vi "MGCC_StaEst_initial_input_RTDS.vi"() -> ()   [LabVIEW 2016]
doc: "-----------------------------------------------------------------------------------------------------------------------\nCopyright <2019> <The University of Tennessee at Knoxville and the University of Tennessee Research Foundation>\nThis software is released under BSD-3 \nhttps://opensource.org/licenses/BSD-3-Clause \nAdditional license options available at https://utrf.tennessee.edu/industry/sample-agreements/\n-----------------------------------------------------------------------------------------------------------------------"
uses:
  <vilib>/Utility/error.llb/Error Cluster From Error Code.vi
  <vilib>/ErrorRing/Error Ring.xnode
panel:
  out "element":i32
  out "size(s)":i32[](array[numeric])
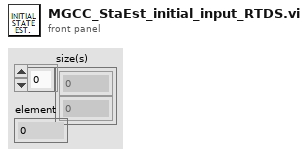
[diagram p1: front panel]
types:
  T1 = cluster{"V_node":cdb[][], "P_node":cdb[][], "I_node":cdb[][], "NumN":dbl, "NumL":dbl, "Ybus":cdb[][], "sspn":dbl[][], "ssqn":dbl[][], "ssvn":dbl[][], "SlackBus":dbl, "Topology":dbl[][]}
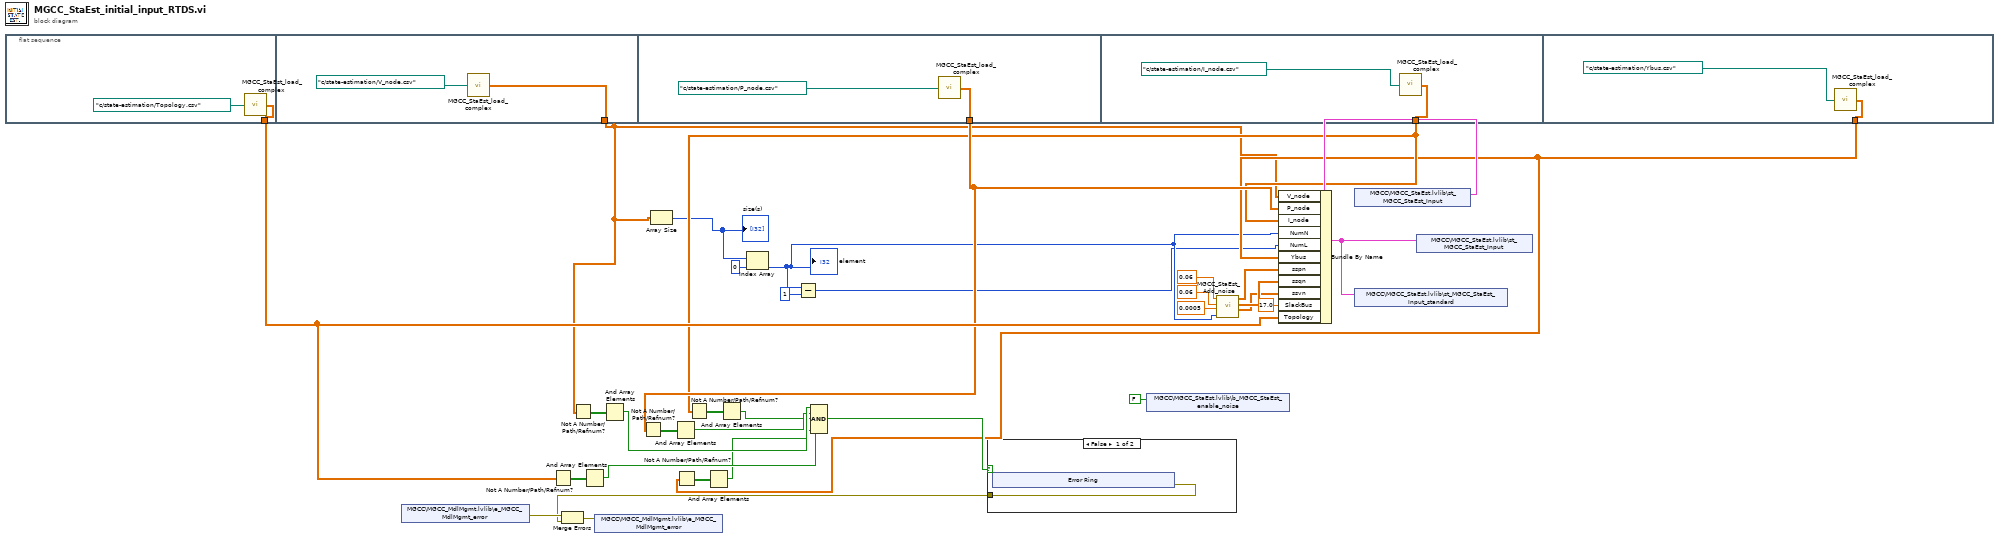
[diagram p0: block diagram]
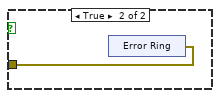
[diagram p2: hidden frame]
diagram:
  n1 = flat-sequence {
    tunnel: [w35] -> w12
    tunnel: [w37] -> w6
    tunnel: [w39] -> w11
    tunnel: [w41] -> w10
    tunnel: [w43] -> w8
    frame #0 {
      n2 = call "MGCC_StaEst_load_complex.vi"("file path (dialog if empty)"=path "c:/state-estimation/Topology.csv" ("file path (use dialog)")) -> ("Array 13"=w35:cdb[][])
    }
    frame #1 {
      n3 = call "MGCC_StaEst_load_complex.vi"("file path (dialog if empty)"=path "c:/state-estimation/V_node.csv" ("file path (use dialog)")) -> ("Array 13"=w37:cdb[][])
    }
    frame #2 {
      n4 = call "MGCC_StaEst_load_complex.vi"("file path (dialog if empty)"=path "c:/state-estimation/P_node.csv" ("file path (use dialog)")) -> ("Array 13"=w39:cdb[][])
    }
    frame #3 {
      n5 = call "MGCC_StaEst_load_complex.vi"("file path (dialog if empty)"=path "c:/state-estimation/I_node.csv" ("file path (use dialog)")) -> ("Array 13"=w41:cdb[][])
    }
    frame #4 {
      n6 = call "MGCC_StaEst_load_complex.vi"("file path (dialog if empty)"=path "c:/state-estimation/Ybus.csv" ("file path (use dialog)")) -> ("Array 13"=w43:cdb[][])
    }
  }
  n7 = shared-variable "MGCC\\MGCC_MdlMgmt.lvlib\\e_MGCC_MdlMgmt_error"() -> (w24:errorcluster)  [unwired: 1 in, 1 out]
  n8 = Not A Number/Path/Refnum?(number/path/refnum=w12) -> (NaN/Path/Refnum?=w21:bool[][])
  n9 = Not A Number/Path/Refnum?(number/path/refnum=w6) -> (NaN/Path/Refnum?=w20:bool[][])
  n10 = And Array Elements(Boolean array=w21) -> (logical AND=w14:bool)
  n11 = And Array Elements(Boolean array=w20) -> (logical AND=w17:bool)
  n12 = Not A Number/Path/Refnum?(number/path/refnum=w11) -> (NaN/Path/Refnum?=w18:bool[][])
  n13 = Array Size(array=w6) -> (size(s)=w5:i32[])
  "size(s)" <- w5
  n14 = And Array Elements(Boolean array=w18) -> (logical AND=w16:bool)
  n15 = Not A Number/Path/Refnum?(number/path/refnum=w8) -> (NaN/Path/Refnum?=w9:bool[][])
  n16 = Not A Number/Path/Refnum?(number/path/refnum=w10) -> (NaN/Path/Refnum?=w19:bool[][])
  n17 = And Array Elements(Boolean array=w9) -> (logical AND=w7:bool)
  n18 = And Array Elements(Boolean array=w19) -> (logical AND=w15:bool)
  n19 = Index Array(array=w5, index=0) -> (element=w2:i32)
  "element" <- w2
  n20 = Subtract(x=w2, y=1) -> (x-y=w1:i32)
  n21 = Compound Arithmetic op=AND(w17, w16, w15, w14, w7) -> (w13:bool)
  n22 = case shown="False" w13 {
    tunnel: [w45 w51] -> w22
    frame False {
      n23 = xnode "Error Ring"() -> ("error out"=w45:errorcluster)
    }
    frame True {
      n24 = xnode "Error Ring"() -> ("error out"=w51:errorcluster)
    }
  }
  n25 = Merge Errors(w24, w22) -> (w23:errorcluster)
  n26 = shared-variable "MGCC\\MGCC_MdlMgmt.lvlib\\e_MGCC_MdlMgmt_error"(w23) -> ()  [unwired: 1 in, 1 out]
  n27 = shared-variable "MGCC\\MGCC_StaEst.lvlib\\b_MGCC_StaEst_enable_noise"(FALSE ("b_MGCC_StaEst_enable_noise")) -> ()  [unwired: 1 in, 1 out]
  n28 = call "MGCC_StaEst_Add_noise.vi"("spn"=0.06, "sqn"=0.06, "svn"=0.0005, "Node"=w2) -> ("sspn"=w27:dbl[][], "ssvn"=w26:dbl[][], "ssqn"=w25:dbl[][])  [unwired: 2 in]
  n29 = shared-variable "MGCC\\MGCC_StaEst.lvlib\\st_MGCC_StaEst_Input"() -> (w32:T1)  [unwired: 1 in, 1 out]
  n30 = Bundle By Name(cluster=w32, "V_node"=w6, "P_node"=w11, "I_node"=w10, "NumN"=w2, "NumL"=w1, "Ybus"=w8, "sspn"=w27, "ssqn"=w26, "ssvn"=w25, "SlackBus"=17.0, "Topology"=w12) -> (w31:T1)
  n31 = shared-variable "MGCC\\MGCC_StaEst.lvlib\\st_MGCC_StaEst_Input_standard"(w31) -> ()  [unwired: 1 in, 1 out]
  n32 = shared-variable "MGCC\\MGCC_StaEst.lvlib\\st_MGCC_StaEst_Input"(w31) -> ()  [unwired: 1 in, 1 out]
